vi "InitializeCore.vi"(8 "error in (no error)":errorcluster, 10 "Connection String":string, 11 "MicronServer in":refnum<class "GRPCService.lvclass">) -> (0 "error out":errorcluster, 2 "MessageUserEvent":refnum<user-event>, 3 "MicronServer out":refnum<class "GRPCService.lvclass">)   [LabVIEW 2019, in "MicronGRPCServer.lvlib" / "GRPCService.lvclass"]
uses:
  GRPCService.lvclass
  Base/Server/Message/MessageBase.lvclass
  GRPCService.lvclass/GRPCService.ctl
  Generated/MicronGRPCGeneratedServer/MicronGRPCGeneratedServer.lvlib
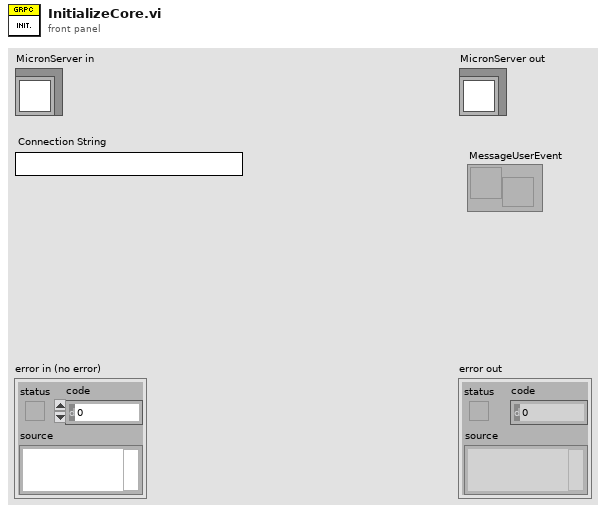
[diagram p1: front panel]
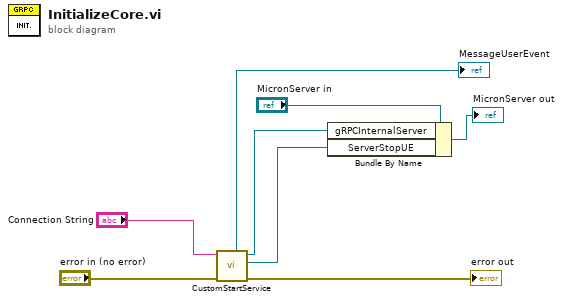
[diagram p0: block diagram]
diagram:
  n1 = call "CustomStartService.vi"("error in"="error in (no error)", "Server Address"="Connection String") -> ("error out"=→"error out":errorcluster, "Server Stop"=w1:refnum<user-event>, "gRPC Server out"=w2:refnum<class "Servicer.lvclass">, "MicronUE"=→"MessageUserEvent":refnum<user-event>)  [unwired: 5 in, 1 out]
  n2 = Bundle By Name(cluster="MicronServer in", "gRPCInternalServer"=w2, "ServerStopUE"=w1) -> (→"MicronServer out":refnum<class "GRPCService.lvclass">)
